vi "Periodic Tasks.vi"(8 "error in":errorcluster) -> ()   [LabVIEW 2018]
doc: "This VI runs in parallel to other robot code. It can contain as many user-defined periodic loops as you need. These can carry out PID or other sorts of timed response."
uses:
  <vilib>/Rock Robotics/WPI/Utilities/WPI_GetSetVariantRefNum.vi
  <vilib>/Rock Robotics/Network Tables/NT Read Number.vi
  <vilib>/Rock Robotics/Network Tables/NT Write Number.vi
  Robot Global Data.vi
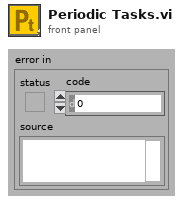
[diagram p1: front panel]
types:
  T1 = typedef "WPI_JoystickDevRef.ctl" = cluster{"Device":T2}
  T2 = typedef "WPI_JoystickDeviceEnum.ctl" = enum16{"USB 0", "USB 1", "USB 2", "USB 3", "USB 4", "USB 5"}
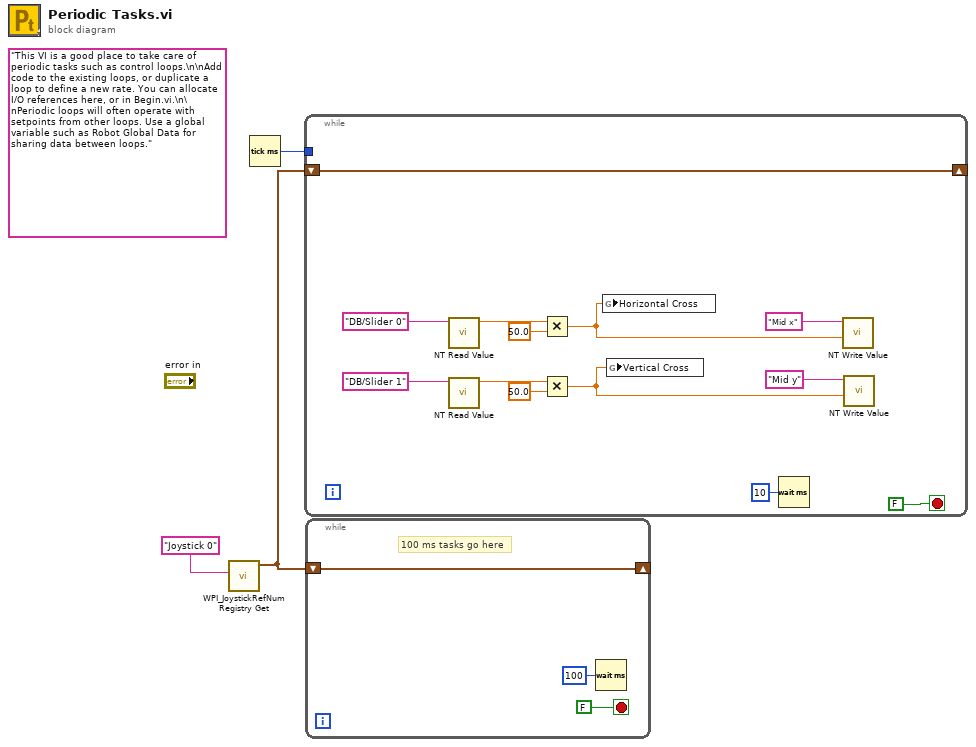
[diagram p0: block diagram]
diagram:
  (unwired) "This VI is a good place to take care of periodic tasks such as control loops.\n\nAdd code to the existing loops, or duplicate a loop to define a new rate. You can allocate I/O references here, or in Begin.vi.\n\nPeriodic loops will often operate with setpoints from other loops. Use a global variable such as Robot Global Data for sharing data between loops."
  n1 = call <vilib>:"WPI_JoystickRefNum Registry Get.vi"("refnum name"="Joystick 0") -> ("JoystickDevRef"=w2:T1)  [unwired: 1 in, 9 out]
  n2 = Tick Count (ms)() -> (millisecond timer value=w1:u32)
  n3 = while {
    shift-right: [w15] -> _
    shift-left: w2 -> [w15]
    tunnel: w1 -> [_]
    stop <- FALSE stop-if-true
    n4 = call-poly <vilib>:"NT Read Value.vi"("Name"="DB/Slider 0") -> ("Numeric"=w6:dbl)  [unwired: 9 in, 1 out]
    n5 = call-poly <vilib>:"NT Read Value.vi"("Name"="DB/Slider 1") -> ("Numeric"=w7:dbl)  [unwired: 9 in, 1 out]
    n6 = Multiply(x=w6, y=50.0) -> (x*y=w5:dbl)
    n7 = Multiply(x=w7, y=50.0) -> (x*y=w4:dbl)
    n8 = global write "Robot Global Data.vi" "Horizontal Cross"(w5) -> ()
    n9 = global write "Robot Global Data.vi" "Vertical Cross"(w4) -> ()
    n10 = Wait (ms)(milliseconds to wait=u32 10) -> ()  [unwired: 1 out]
    n11 = call-poly <vilib>:"NT Write Value.vi"("Numeric"=w5, "Name"="Mid x") -> ()  [unwired: 9 in, 1 out]
    n12 = call-poly <vilib>:"NT Write Value.vi"("Numeric"=w4, "Name"="Mid y") -> ()  [unwired: 9 in, 1 out]
  }
  n13 = while {
    shift-right: [w17] -> _
    shift-left: w2 -> [w17]
    stop <- FALSE stop-if-true
    # "100 ms tasks go here"
    n14 = Wait (ms)(milliseconds to wait=u32 100) -> ()  [unwired: 1 out]
  }
